vi "filter.post.state.vi"(11 "filter.data in":T1 {"get.state"."v"."Quantity" format="%.0x"; "get.state"."v"."OrderId" format="%.0x"; "mem.cmd"."ord.2"."v"."Quantity" format="%016x"; "mem.cmd"."ord.2"."v"."OrderId" format="%016x"; "mem.cmd"."ord.1"."v"."Quantity" format="%016x"; "mem.cmd"."ord.1"."v"."OrderId" format="%016x"; "mem.cmd"."ticker"."v"."Symbol" format="%016x"; "mem.cmd"."order.slot.value"."Quantity" format="%016x"; "mem.cmd"."order.slot.value"."OrderId" format="%016x"; "debug"."v"."slot.3" format="%.0x"; "debug"."v"."slot.2" format="%.0x"; "debug"."v"."slot.1" format="%.0x"; "debug"."v"."slot.0" format="%.0x"; "Scratch"."OrderId" format="%016x"; "hash.2"."data.in" format="%.0x"; "hash.2"."crc32.out" format="%.0x"; "hash.1"."data.in" format="%.0x"; "hash.1"."crc32.out" format="%.0x"}) -> (3 "filter.data out 2":T1 {"get.state"."v"."Quantity" format="%.0x"; "get.state"."v"."OrderId" format="%.0x"; "mem.cmd"."ord.2"."v"."Quantity" format="%016x"; "mem.cmd"."ord.2"."v"."OrderId" format="%016x"; "mem.cmd"."ord.1"."v"."Quantity" format="%016x"; "mem.cmd"."ord.1"."v"."OrderId" format="%016x"; "mem.cmd"."ticker"."v"."Symbol" format="%016x"; "mem.cmd"."order.slot.value"."Quantity" format="%016x"; "mem.cmd"."order.slot.value"."OrderId" format="%016x"; "debug"."v"."slot.3" format="%.0x"; "debug"."v"."slot.2" format="%.0x"; "debug"."v"."slot.1" format="%.0x"; "debug"."v"."slot.0" format="%.0x"; "Scratch"."OrderId" format="%016x"; "hash.2"."data.in" format="%.0x"; "hash.2"."crc32.out" format="%.0x"; "hash.1"."data.in" format="%.0x"; "hash.1"."crc32.out" format="%.0x"})   [LabVIEW 2020]
uses:
  <vilib>/rvi/LocalResourceManager/LocalResourceManager.xnode
  <vilib>/rvi/eio/common/nirviEmuReportErrorAndStop.vi
  <vilib>/rvi/DataTransferAndStorage/Container/Common/niFpgaContainerGetUniqueNameForEmu.vi
  <vilib>/rvi/DataTransferAndStorage/Container/Common/niFpgaContainerSetEmuInfo.vi
  <vilib>/rvi/DataTransferAndStorage/Container/XNode/niFpgaContainer.xnode
  <vilib>/rvi/Memory/Memory_Emulation/niFpgaMemoryEmulationRefIn.vi
  <vilib>/rvi/FIFO/Fifo_Resource/nirvififoEmulationWrite.vi
  Market.Data.Common/fpga/fpganow.common.fpga.lvlib
  filter.debug.slot.ctl
  filter.debug.ctl
  filter.state.slot.ctl
  filter.state.ctl
  filter.states.ctl
  filter.data.scratch.ctl
  Market.Data.Common/fpga/orderbook.command.ctl
  ticker.slot.ctl
  order.slot.ctl
  filter.memory.command.ctl
  filter.data.ctl
  Market.Data.Common/fpga/orderbook.command.type.ctl
  order.slot.hm.ctl
  filter.hash.ctl
  ticker.slot.access.ctl
  order.slot.access.ctl
  Filter.lvclass
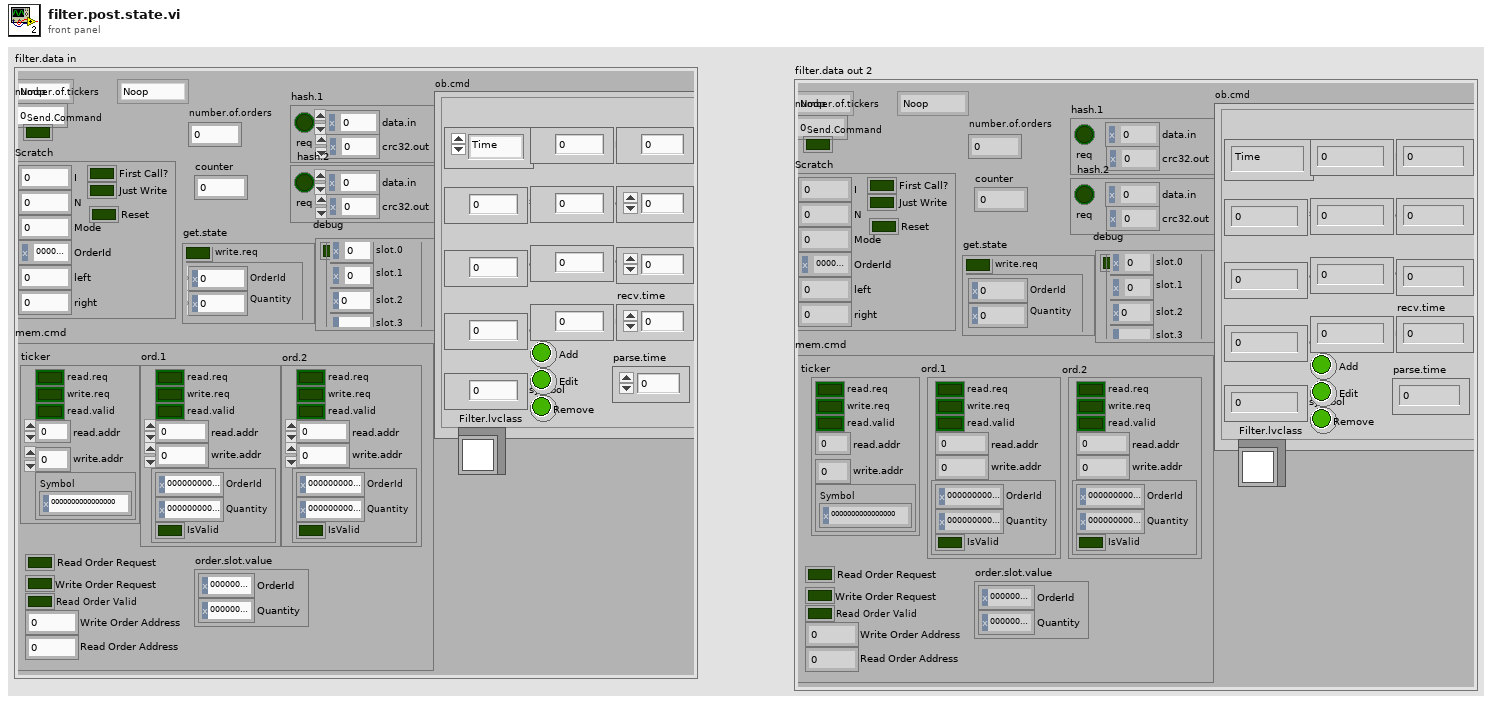
[diagram p1: front panel]
types:
  T1 = typedef "filter.data.ctl" = cluster{"filter.state":T2, "number.of.tickers":u32, "filter.saved.state":T2, "Send.Command":bool, "hash.1":T3, "hash.2":T3, "Scratch":T4, "debug":T5, "mem.cmd":T7, "get.state":T13, "ob.cmd":T15, "number.of.orders":u32, "Filter.lvclass":refnum<class "Filter.lvclass">, "counter":i16}
  T2 = typedef "filter.states.ctl" = enum16{"Noop", "Reset", "Debug", "Configuration", "Wait.for.Command", "Filter.Add", "Filter.Other", "Insert.Order", "Delete Order", "Get.State", "Get.Watchlist", "Get.Memory"}
  T3 = typedef "filter.hash.ctl" = cluster{"req":bool, "data.in":u64, "crc32.out":u32}
  T4 = typedef "filter.data.scratch.ctl" = cluster{"I":u32, "N":u32, "Mode":u32, "OrderId":u64, "First Call?":bool, "Just Write":bool, "left":u32, "right":u32, "Reset":bool}
  T5 = typedef "filter.debug.ctl" = cluster{"write":bool, "v":T6}
  T6 = typedef "filter.debug.slot.ctl" = cluster{"slot.0":u64, "slot.1":u64, "slot.2":u64, "slot.3":u64}
  T7 = typedef "filter.memory.command.ctl" = cluster{"Read Order Request":bool, "Write Order Request":bool, "Read Order Valid":bool, "Write Order Address":u32, "Read Order Address":u32, "order.slot.value":T8, "ticker":T9, "ord.1":T11, "ord.2":T11}
  T8 = typedef "order.slot.ctl" = cluster{"OrderId":u64, "Quantity":u64}
  T9 = typedef "ticker.slot.access.ctl" = cluster{"read.req":bool, "write.req":bool, "read.valid":bool, "read.addr":u32, "write.addr":u32, "v":T10}
  T10 = typedef "ticker.slot.ctl" = cluster{"Symbol":u64}
  T11 = typedef "order.slot.access.ctl" = cluster{"read.req":bool, "write.req":bool, "read.valid":bool, "read.addr":u32, "write.addr":u32, "v":T12}
  T12 = typedef "order.slot.hm.ctl" = cluster{"OrderId":u64, "Quantity":u64, "IsValid":bool}
  T13 = typedef "filter.state.ctl" = cluster{"write.req":bool, "v":T14}
  T14 = typedef "filter.state.slot.ctl" = cluster{"OrderId":u64, "Quantity":u64}
  T15 = typedef "fpganow.common.fpga.lvlib/orderbook.command.ctl" = cluster{"type":T16, "side":u8, "orderId ":u64, "quantity":u32, "symbol":u64, "price":u64, "executed.qty":u32, "canceled.qty":u32, "remaining.qty":u32, "seconds":u64, "nanoseconds":u64, "Add":bool, "Edit":bool, "Remove":bool, "seq no":u32, "recv.time":u64, "parse.time":u64}
  T16 = typedef "fpganow.common.fpga.lvlib/orderbook.command.type.ctl" = enum8{"Time", "AddOrder", "OrderExecuted", "OrderExecutedAtPrice", "ReduceSize", "ModifyOrder", "DeleteOrder", "Get.Everything", "Get.All.Orders", "Get.Top"}
  T17 = cluster{"OrderId":u64, "Quantity":u64, "IsValid":bool}
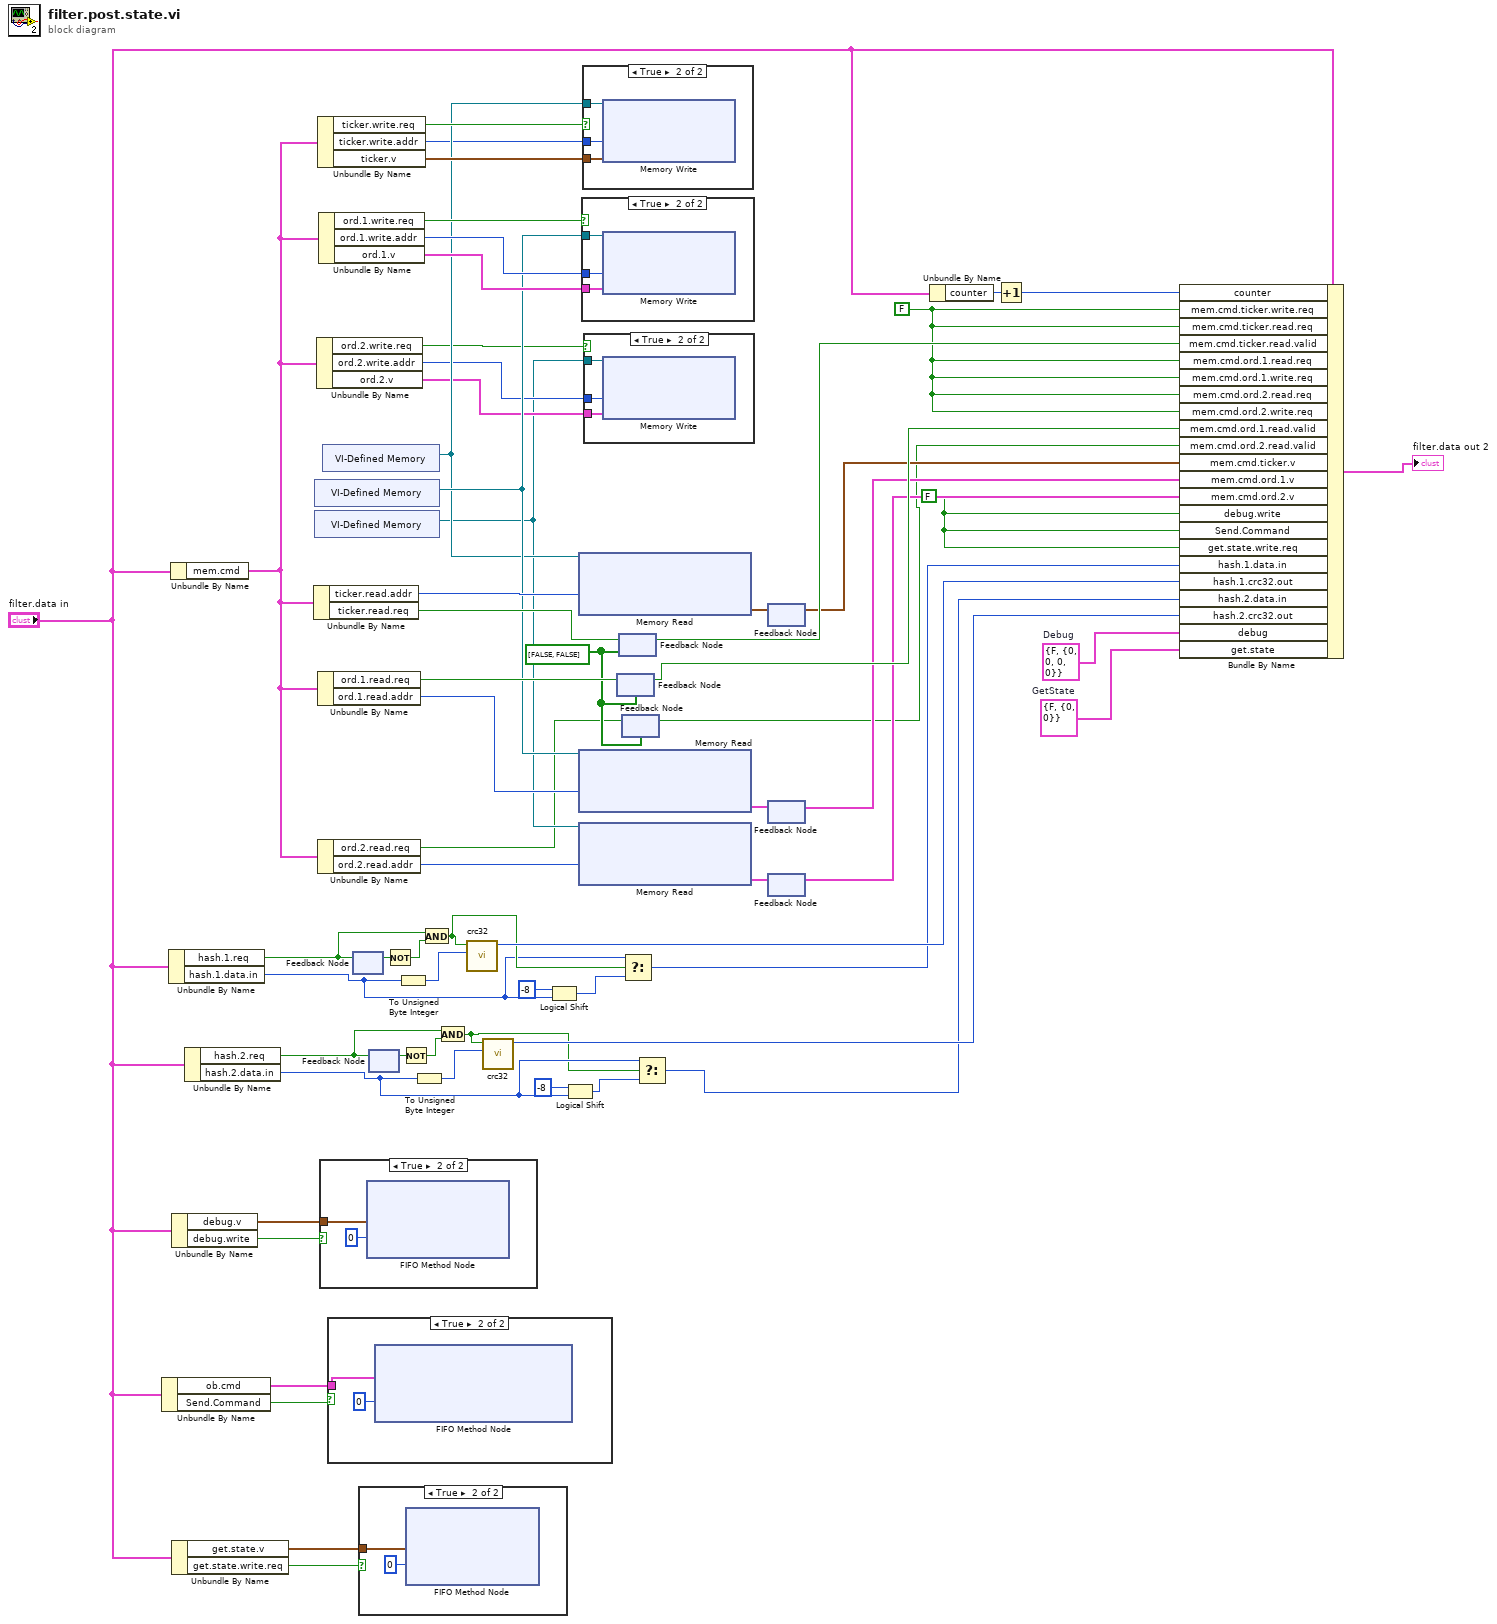
[diagram p0: block diagram]
diagram:
  w13 = T13 {"write.req"=FALSE, "v"={"OrderId"=0, "Quantity"=0}}  # GetState
  w14 = T5 {"write"=FALSE, "v"={"slot.0"=0, "slot.1"=0, "slot.2"=0, "slot.3"=0}}  # Debug
  w4 = FALSE ("memory.command.Write Ticker\nRequest")
  w32 = bool[] [FALSE, FALSE]
  w29 = FALSE ("Debug.Write.to.Debug")
  n1 = Unbundle By Name("filter.data in") -> ("ob.cmd"=w53:T15, "Send.Command"=w52:bool)
  n2 = Unbundle By Name("filter.data in") -> ("hash.1.req"=w26:bool, "hash.1.data.in"=w11:u64)
  n3 = Unbundle By Name("filter.data in") -> ("mem.cmd"=w27:T7)
  n4 = Unbundle By Name("filter.data in") -> ("debug.v"=w51:T6, "debug.write"=w49:bool)
  n5 = Unbundle By Name("filter.data in") -> ("get.state.v"=w39:T14, "get.state.write.req"=w40:bool)
  n6 = Unbundle By Name("filter.data in") -> ("hash.2.req"=w20:bool, "hash.2.data.in"=w8:u64)
  n7 = Unbundle By Name(w27) -> ("ticker.read.addr"=w44:u32, "ticker.read.req"=w59:bool)
  n8 = xnode "VI-Defined Memory"() -> ("Memory Out"=w43:refnum<k21>)
  n9 = xnode "VI-Defined Memory"() -> ("Memory Out"=w35:refnum<k21>)
  n10 = Unbundle By Name(w27) -> ("ord.2.write.req"=w36:bool, "ord.2.write.addr"=w38:u32, "ord.2.v"=w37:T12)
  n11 = Unbundle By Name(w27) -> ("ticker.write.req"=w54:bool, "ticker.write.addr"=w41:u32, "ticker.v"=w55:T10)
  n12 = Unbundle By Name(w27) -> ("ord.1.read.req"=w61:bool, "ord.1.read.addr"=w60:u32)
  n13 = Unbundle By Name(w27) -> ("ord.2.read.req"=w31:bool, "ord.2.read.addr"=w33:u32)
  n14 = Unbundle By Name(w27) -> ("ord.1.write.req"=w56:bool, "ord.1.write.addr"=w57:u32, "ord.1.v"=w58:T12)
  n15 = case shown="True" w49 {
    tunnel: w51 -> [_ w65]
    frame False {
    }
    frame True {
      n16 = xnode ("FIFO Method Node")("Element"=w65, "Timeout"=0) -> ()  [unwired: 1 in, 2 out]
    }
  }
  n17 = xnode "VI-Defined Memory"() -> ("Memory Out"=w42:refnum<k21>)
  n18 = case shown="True" w52 {
    tunnel: w53 -> [_ w66]
    frame False {
    }
    frame True {
      n19 = xnode ("FIFO Method Node")("Element"=w66, "Timeout"=0) -> ()  [unwired: 1 in, 2 out]
    }
  }
  n20 = feedback-in #1(w26) -> ()
  n21 = feedback #1() -> (w25:bool)  [unwired: 1 in]
  n22 = case shown="True" w40 {
    tunnel: w39 -> [_ w69]
    frame False {
    }
    frame True {
      n23 = xnode ("FIFO Method Node")("Element"=w69, "Timeout"=0) -> ()  [unwired: 1 in, 2 out]
    }
  }
  n24 = feedback #2() -> (w19:bool)  [unwired: 1 in]
  n25 = feedback-in #2(w20) -> ()
  n26 = Not(x=w25) -> (.not. x?=w24:bool)
  n27 = To Unsigned Byte Integer(number=w11) -> (unsigned 8bit integer=w23:u8)
  n28 = Not(x=w19) -> (.not. x?=w18:bool)
  n29 = To Unsigned Byte Integer(number=w8) -> (unsigned 8bit integer=w17:u8)
  n30 = And(x=w26, y=w24) -> (x .and. y?=w12:bool)
  n31 = And(x=w20, y=w18) -> (x .and. y?=w5:bool)
  n32 = call "crc32.vi"("Data.in"=w23, "Reset"=w12) -> ("CRC32.out"=w22:u32)  [unwired: 9 in]
  n33 = call "crc32.vi"("Data.in"=w17, "Reset"=w5) -> ("CRC32.out"=w15:u32)  [unwired: 9 in]
  n34 = Logical Shift(y=i16 -8, x=w11) -> (x << y=w10:u64)
  n35 = Logical Shift(y=i16 -8, x=w8) -> (x << y=w6:u64)
  n36 = xnode "Memory Read"("Address"=w44, "Memory In"=w42) -> ("Data"=w46:cluster{"Symbol":u64})  [unwired: 1 out]
  n37 = xnode "Memory Read"("Address"=w60, "Memory In"=w43) -> ("Data"=w45:T17)  [unwired: 1 out]
  n38 = xnode "Memory Read"("Address"=w33, "Memory In"=w35) -> ("Data"=w34:T17)  [unwired: 1 out]
  n39 = case shown="True" w56 {
    tunnel: w43 -> [_ w72]
    tunnel: w57 -> [_ w71]
    tunnel: w58 -> [_ w70]
    frame False {
    }
    frame True {
      n40 = xnode "Memory Write"("Address"=w71, "Data"=w70, "Memory In"=w72) -> ()  [unwired: 1 out]
    }
  }
  n41 = case shown="True" w54 {
    tunnel: w42 -> [_ w75]
    tunnel: w41 -> [_ w74]
    tunnel: w55 -> [_ w73]
    frame False {
    }
    frame True {
      n42 = xnode "Memory Write"("Address"=w74, "Data"=w73, "Memory In"=w75) -> ()  [unwired: 1 out]
    }
  }
  n43 = case shown="True" w36 {
    tunnel: w35 -> [_ w78]
    tunnel: w38 -> [_ w77]
    tunnel: w37 -> [_ w76]
    frame False {
    }
    frame True {
      n44 = xnode "Memory Write"("Address"=w77, "Data"=w76, "Memory In"=w78) -> ()  [unwired: 1 out]
    }
  }
  n45 = feedback #3(w32) -> (w63:bool)
  n46 = feedback-in #3(w61) -> ()
  n47 = feedback #4(w32) -> (w62:bool)
  n48 = feedback-in #4(w59) -> ()
  n49 = feedback #5(w32) -> (w28:bool)
  n50 = feedback-in #5(w31) -> ()
  n51 = Select(t=w11, s=w12, f=w10) -> (s? t:f=w9:u64)
  n52 = Select(t=w8, s=w5, f=w6) -> (s? t:f=w7:u64)
  n53 = feedback #6() -> (w50:cluster{"Symbol":u64})  [unwired: 1 in]
  n54 = feedback-in #6(w46) -> ()
  n55 = feedback #7() -> (w48:T17)  [unwired: 1 in]
  n56 = feedback-in #7(w45) -> ()
  n57 = feedback #8() -> (w30:T17)  [unwired: 1 in]
  n58 = feedback-in #8(w34) -> ()
  n59 = Unbundle By Name("filter.data in") -> ("counter"=w2:i16)
  n60 = Increment(x=w2) -> (x+1=w1:i16)
  n61 = Bundle By Name(cluster="filter.data in", "counter"=w1, "mem.cmd.ticker.write.req"=w4, "mem.cmd.ticker.read.req"=w4, "mem.cmd.ticker.read.valid"=w62, "mem.cmd.ord.1.read.req"=w4, "mem.cmd.ord.1.write.req"=w4, "mem.cmd.ord.2.read.req"=w4, "mem.cmd.ord.2.write.req"=w4, "mem.cmd.ord.1.read.valid"=w63, "mem.cmd.ord.2.read.valid"=w28, "mem.cmd.ticker.v"=w50, "mem.cmd.ord.1.v"=w48, "mem.cmd.ord.2.v"=w30, "debug.write"=w29, "Send.Command"=w29, "get.state.write.req"=w29, "hash.1.data.in"=w9, "hash.1.crc32.out"=w22, "hash.2.data.in"=w7, "hash.2.crc32.out"=w15, "debug"=w14, "get.state"=w13) -> (→"filter.data out 2":T1)
